vi "PathPlanner_Trajectory_GenerateStates_Pass1.vi"(9 "StartingSpeeds":T5 {"vOmega" format="%10.3f"; "vY" format="%10.3f"; "vX" format="%10.3f"}, 10 "in PathPlannerStates":T1[](array[typedef]) {"TargetHolonomicRotation"."SIN" format="%13.4f"; "TargetHolonomicRotation"."COS" format="%13.4f"; "TargetHolonomicRotation"."VALUE" format="%13.4f"; "Heading"."SIN" format="%13.4f"; "Heading"."COS" format="%13.4f"; "Heading"."VALUE" format="%13.4f"; "PositionMeters"."Y" format="%14.3f"; "PositionMeters"."X" format="%14.3f"}, 11 "PathPlannerPath":T6={"Reversed"=FALSE, "RotationTargets"=[], "ConstraintZones"=[], "EventMarkers"=[], "GlobalConstraints"={"MaxVelocityMps;"=0.0, "MaxAccelerationMpsSq;"=0.0, "MaxAngularVelRadPsEc;"=0.0, "MaxAngularAccRadPSecSq"=0.0, "Exists"=FALSE, "Unlimited"=FALSE, "NominalVoltageVolts"=12.0}, "GoalEndState"={"VelocityMPS"=0.0, "Rotation"={"VALUE"=0.0, "COS"=1.0, "SIN"=0.0}}, "AllPoints"=[], "Name"="", "Waypoints"=[], "PointTowardsZones"=[], "IdealStartingState"={"VelocityMPS"=0.0, "Rotation"={"VALUE"=1.0, "COS"=0.0, "SIN"=0.0}}, "IsChoreoPath"=FALSE, "PreventFlipping"=FALSE} {"IdealStartingState"."Rotation"."SIN" format="%13.4f"; "IdealStartingState"."Rotation"."COS" format="%13.4f"; "IdealStartingState"."Rotation"."VALUE" format="%13.4f"; "PointTowardsZones"."TargetPosition"."Y" format="%14.3f"; "PointTowardsZones"."TargetPosition"."X" format="%14.3f"; "PointTowardsZones"."RotationOffset"."SIN" format="%13.4f"; "PointTowardsZones"."RotationOffset"."COS" format="%13.4f"; "PointTowardsZones"."RotationOffset"."VALUE" format="%13.4f"; "Waypoints"."nextControl"."Y" format="%14.3f"; "Waypoints"."nextControl"."X" format="%14.3f"; "Waypoints"."anchor"."Y" format="%14.3f"; "Waypoints"."anchor"."X" format="%14.3f"; "Waypoints"."prevControl"."Y" format="%14.3f"; "Waypoints"."prevControl"."X" format="%14.3f"; "AllPoints"."RotationTarget"."rotation"."SIN" format="%13.4f"; "AllPoints"."RotationTarget"."rotation"."COS" format="%13.4f"; "AllPoints"."RotationTarget"."rotation"."VALUE" format="%13.4f"; "AllPoints"."Position"."Y" format="%14.3f"; "AllPoints"."Position"."X" format="%14.3f"; "GoalEndState"."Rotation"."SIN" format="%13.4f"; "GoalEndState"."Rotation"."COS" format="%13.4f"; "GoalEndState"."Rotation"."VALUE" format="%13.4f"; "RotationTargets"."rotation"."SIN" format="%13.4f"; "RotationTargets"."rotation"."COS" format="%13.4f"; "RotationTargets"."rotation"."VALUE" format="%13.4f"}) -> (3 "out PathPlannerStates":T1[](array[typedef]) {"TargetHolonomicRotation"."SIN" format="%13.4f"; "TargetHolonomicRotation"."COS" format="%13.4f"; "TargetHolonomicRotation"."VALUE" format="%13.4f"; "Heading"."SIN" format="%13.4f"; "Heading"."COS" format="%13.4f"; "Heading"."VALUE" format="%13.4f"; "PositionMeters"."Y" format="%14.3f"; "PositionMeters"."X" format="%14.3f"})   [LabVIEW 2019, in "PathPlanner24.lvlib"]
doc: "Internal routine to help create a trajectory from a path."
uses:
  PathPlanner24.lvlib
  TypeDef/PathPlannerTrajectoryState.ctl
  <vilib>/Rock Robotics/WPI/ThirdParty/JAS_Junk/TrajLib/TypeDef/TRANSLATION2D.ctl
  <vilib>/Rock Robotics/WPI/ThirdParty/JAS_Junk/TrajLib/TypeDef/ROTATION2D.ctl
  TypeDef/PathPlannerPathConstraints.ctl
  TypeDef/PathPlannerPath.ctl
  TypeDef/PathPlannerRotationTarget.ctl
  TypeDef/PathPlannerConstraintsZone.ctl
  TypeDef/PathPlannerEventMarker.ctl
  TypeDef/PathPlannerCommandUtil.ctl
  ENum/PathPlanner_CommandUtilType_ENUM.ctl
  TypeDef/PathPlannerGoalEndState.ctl
  TypeDef/PathPlannerPathPoint.ctl
  TypeDef/PathPlannerWaypoint.ctl
  TypeDef/PathPlannerPointTowardsZone.ctl
  TypeDef/PathPlannerIdealStartingState.ctl
  <vilib>/Rock Robotics/WPI/ThirdParty/JAS_Junk/TrajLib/TypeDef/CHASSIS_SPEEDS.ctl
  PathPlanner_GeomUtil_CalculateRadius.vi
  <vilib>/Rock Robotics/WPI/ThirdParty/JAS_Junk/TrajLib/Translation2d_Create.vi
  <vilib>/Rock Robotics/WPI/ThirdParty/JAS_Junk/TrajLib/Translation2d_GetXY.vi
  <vilib>/Rock Robotics/WPI/ThirdParty/JAS_Junk/TrajLib/Rotation2d_CreateXY.vi
  <vilib>/Rock Robotics/WPI/ThirdParty/JAS_Junk/TrajLib/Translation2d_GetDistance.vi
  <vilib>/Rock Robotics/WPI/ThirdParty/JAS_Junk/TrajLib/Trajectory_Library.lvlib
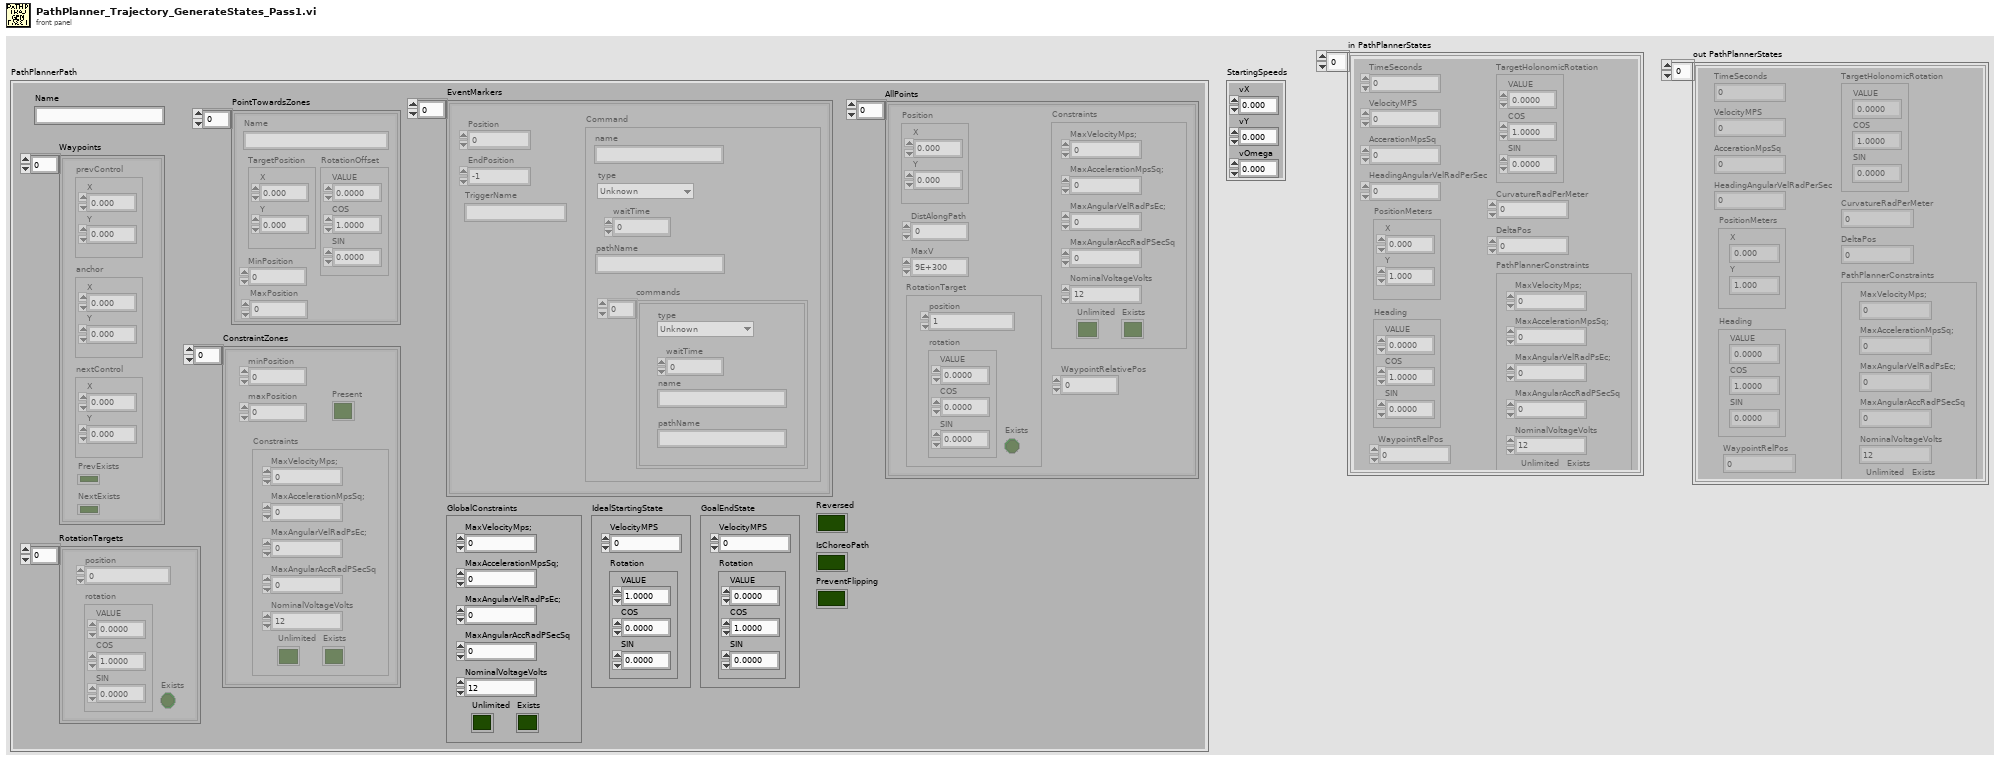
[diagram p1: front panel]
types:
  T1 = typedef "PathPlanner24.lvlib/PathPlannerTrajectoryState.ctl" = cluster{"TimeSeconds":dbl, "VelocityMPS":dbl, "AccerationMpsSq":dbl, "HeadingAngularVelRadPerSec":dbl, "PositionMeters":T2, "Heading":T3, "TargetHolonomicRotation":T3, "CurvatureRadPerMeter":dbl, "PathPlannerConstraints":T4, "DeltaPos":dbl, "WaypointRelPos":dbl}
  T2 = typedef "Trajectory_Library.lvlib/TRANSLATION2D.ctl" = cluster{"X":dbl, "Y":dbl}
  T3 = typedef "Trajectory_Library.lvlib/ROTATION2D.ctl" = cluster{"VALUE":dbl, "COS":dbl, "SIN":dbl}
  T4 = typedef "PathPlanner24.lvlib/PathPlannerPathConstraints.ctl" = cluster{"MaxVelocityMps;":dbl, "MaxAccelerationMpsSq;":dbl, "MaxAngularVelRadPsEc;":dbl, "MaxAngularAccRadPSecSq":dbl, "Exists":bool, "Unlimited":bool, "NominalVoltageVolts":dbl}
  T5 = typedef "Trajectory_Library.lvlib/CHASSIS_SPEEDS.ctl" = cluster{"vX":dbl, "vY":dbl, "vOmega":dbl}
  T6 = typedef "PathPlanner24.lvlib/PathPlannerPath.ctl" = cluster{"Reversed":bool, "RotationTargets":T7[], "ConstraintZones":T8[], "EventMarkers":T9[], "GlobalConstraints":T4, "GoalEndState":T12, "AllPoints":T13[], "Name":string, "Waypoints":T14[], "PointTowardsZones":T15[], "IdealStartingState":T16, "IsChoreoPath":bool, "PreventFlipping":bool}
  T7 = typedef "PathPlanner24.lvlib/PathPlannerRotationTarget.ctl" = cluster{"position":dbl, "rotation":T3, "Exists":bool}
  T8 = typedef "PathPlanner24.lvlib/PathPlannerConstraintsZone.ctl" = cluster{"minPosition":dbl, "maxPosition":dbl, "Constraints":T4, "Present":bool}
  T9 = typedef "PathPlanner24.lvlib/PathPlannerEventMarker.ctl" = cluster{"Position":dbl, "Command":T10, "TriggerName":string, "EndPosition":dbl}
  T10 = typedef "PathPlanner24.lvlib/PathPlannerCommandUtil.ctl" = cluster{"waitTime":dbl, "name":string, "pathName":string, "commands":cluster{"type":T11, "waitTime":dbl, "name":string, "pathName":string}[], "type":T11}
  T11 = typedef "PathPlanner24.lvlib/PathPlanner_CommandUtilType_ENUM.ctl" = enum16{"Unknown", "Wait", "Named", "Path", "Sequential", "Parallel", "Race", "Deadline"}
  T12 = typedef "PathPlanner24.lvlib/PathPlannerGoalEndState.ctl" = cluster{"VelocityMPS":dbl, "Rotation":T3}
  T13 = typedef "PathPlanner24.lvlib/PathPlannerPathPoint.ctl" = cluster{"Position":T2, "DistAlongPath":dbl, "MaxV":dbl, "Constraints":T4, "RotationTarget":T7, "WaypointRelativePos":dbl}
  T14 = typedef "PathPlanner24.lvlib/PathPlannerWaypoint.ctl" = cluster{"prevControl":T2, "anchor":T2, "nextControl":T2, "PrevExists":bool, "NextExists":bool}
  T15 = typedef "PathPlanner24.lvlib/PathPlannerPointTowardsZone.ctl" = cluster{"RotationOffset":T3, "Name":string, "TargetPosition":T2, "MinPosition":dbl, "MaxPosition":dbl}
  T16 = typedef "PathPlanner24.lvlib/PathPlannerIdealStartingState.ctl" = cluster{"VelocityMPS":dbl, "Rotation":T3}
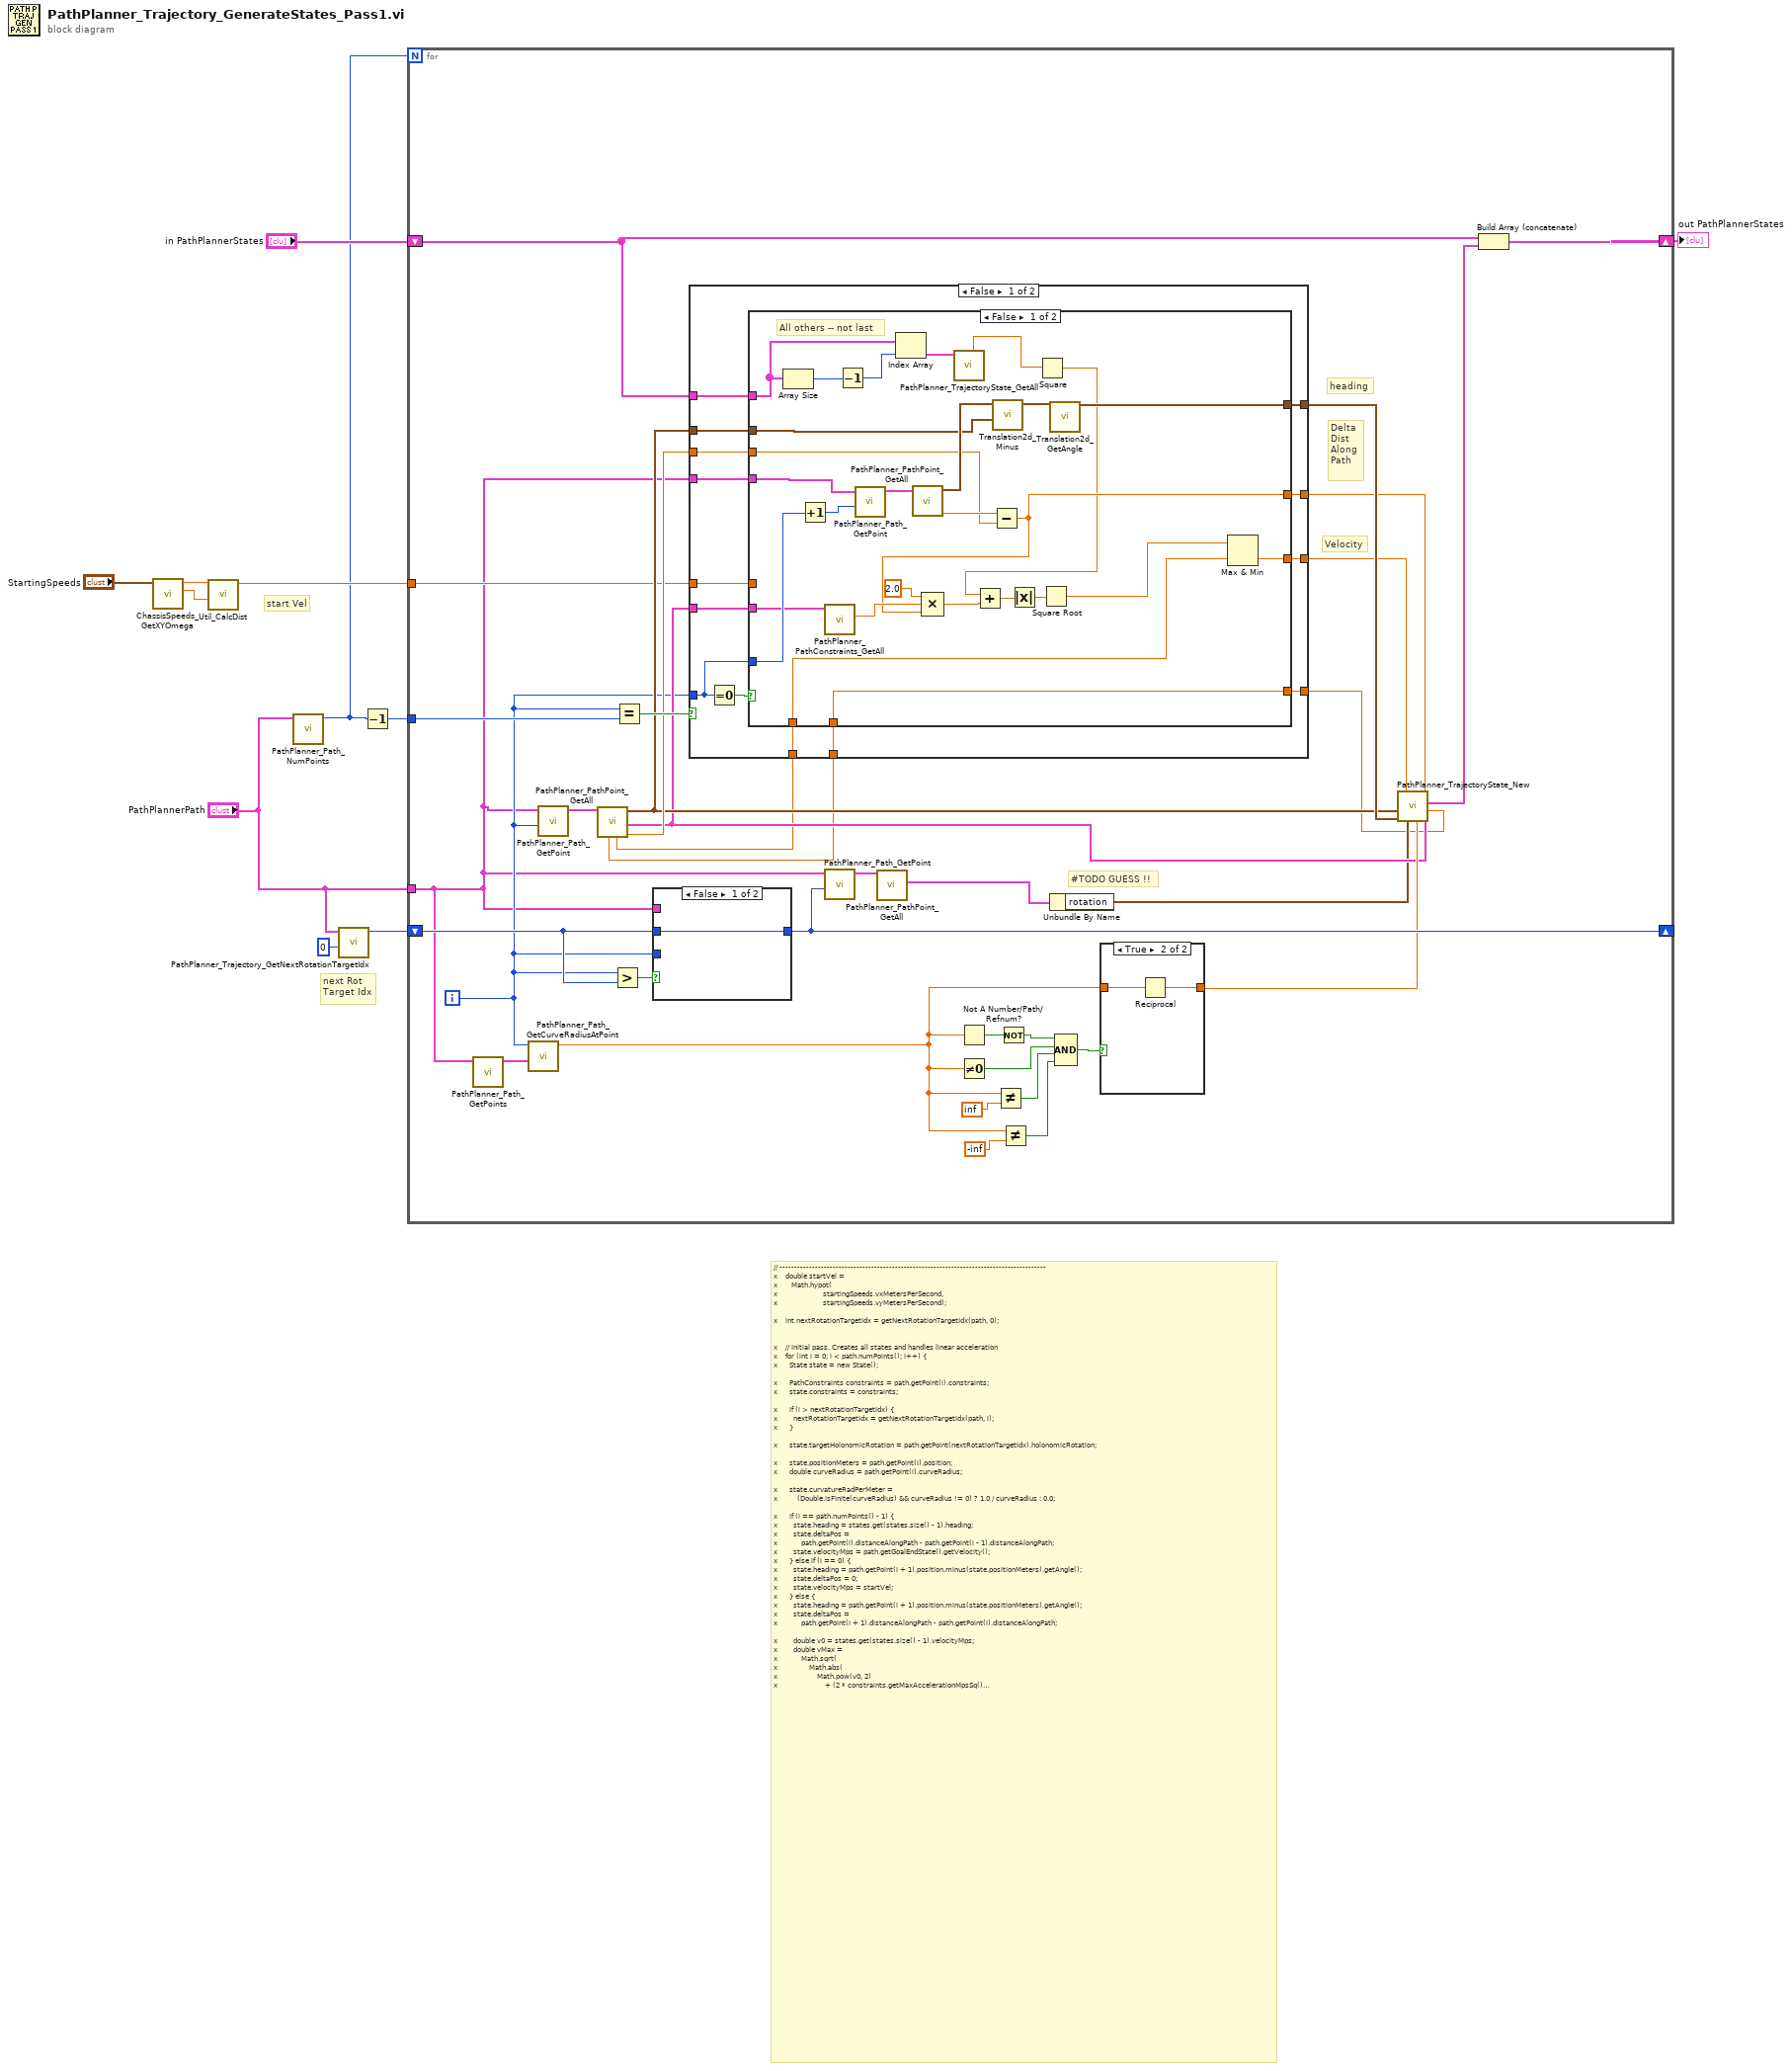
[diagram p0: block diagram]
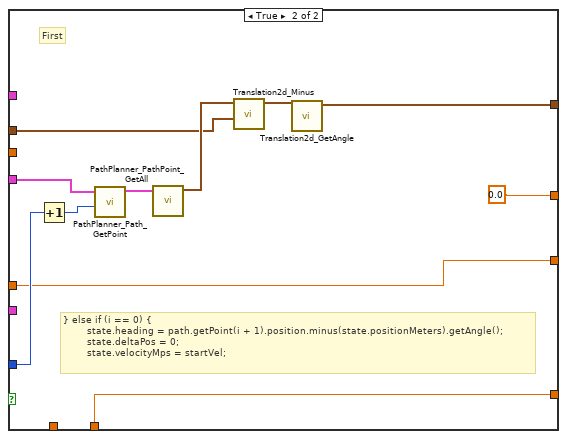
[diagram p2: hidden frame]
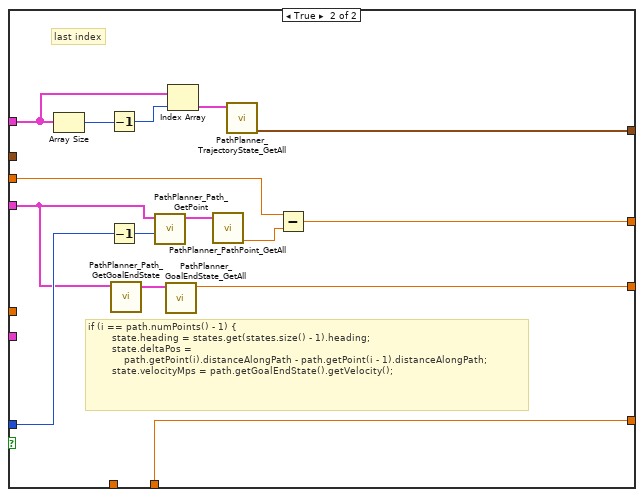
[diagram p3: hidden frame]
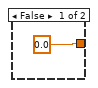
[diagram p4: hidden frame]
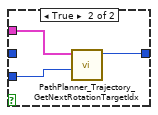
[diagram p5: hidden frame]
diagram:
  # "next Rot\nTarget Idx"
  # "start Vel"
  # "// ------------------------------------------------------------------------------------------\nx    double startVel =\nx       Math.hypot(  \nx                       startingSpeeds.vxMetersPerSecond, \nx                       startingSpeeds.vyMetersPerSecond);\n\nx    int nextRotationTargetIdx = getNextRotationTargetIdx(path, 0);\n\n\nx    // Initial pass. Creates all states and handles linear acceleration\nx    for (int i = 0; i < path.numPoints(); i++) {\nx      State state = new State();\n\nx      PathConstraints constraints = path.getPoint(i).constraints;\nx      state.constraints = constraints;\n\nx      if (i > nextRotationTargetIdx) {\nx        nextRotationTargetIdx = getNextRotationTargetIdx(path, i);\nx      }\n\nx      state.targetHolonomicRotation = path.getPoint(nextRotationTargetIdx).holonomicRotation;\n\nx      state.positionMeters = path.getPoint(i).position;\nx      double curveRadius = path.getPoint(i).curveRadius;\n\nx      state.curvatureRadPerMeter =\nx          (Double.isFinite(curveRadius) && curveRadius != 0) ? 1.0 / curveRadius : 0.0;\n\nx      if (i == path.numPoints() - 1) {\nx        state.heading = states.get(states.size() - 1).heading;\nx        state.deltaPos =\nx            path.getPoint(i).distanceAlongPath - path.getPoint(i - 1).distanceAlongPath;\nx        state.velocityMps = path.getGoalEndState().getVelocity();\nx      } else if (i == 0) {\nx        state.heading = path.getPoint(i + 1).position.minus(state.positionMeters).getAngle();\nx        state.deltaPos = 0;\nx        state.velocityMps = startVel;\nx      } else {\nx        state.heading = path.getPoint(i + 1).position.minus(state.positionMeters).getAngle();\nx        state.deltaPos =\nx            path.getPoint(i + 1).distanceAlongPath - path.getPoint(i).distanceAlongPath;\n\nx        double v0 = states.get(states.size() - 1).velocityMps;\nx        double vMax =\nx            Math.sqrt(\nx                Math.abs(\nx                    Math.pow(v0, 2)\nx                        + (2 * constraints.getMaxAccelerationMpsSq() * state.deltaPos)));\nx        state.velocityMps = Math.min(vMax, path.getPoint(i).maxV);\n      }\n\nX      states.add(state);\n    }"
  n1 = call <vilib>:"ChassisSpeeds_GetXYOmega.vi"("CHASSIS"="StartingSpeeds") -> ("vY"=w5:dbl, "vX"=w6:dbl)  [unwired: 8 in, 1 out]
  n2 = call <vilib>:"Util_CalcDist.vi"("Y"=w5, "X"=w6) -> ("DIST"=w4:dbl)  [unwired: 9 in]
  n3 = call "PathPlanner_Path_NumPoints.vi"("PathPlannerPath"="PathPlannerPath") -> ("NumPoints"=w1:i32)  [unwired: 10 in]
  n4 = call "PathPlanner_Trajectory_GetNextRotationTargetIdx.vi"("Starting Index"=0, "PathPlannerPath"="PathPlannerPath") -> ("Idx"=w8:i32)  [unwired: 8 in, 1 out]
  n5 = Decrement(x=w1) -> (x-1=w3:i32)
  n6 = for {
    N: w1 -> [_]
    shift-right: [w46] -> w10
    shift-left: "in PathPlannerStates" -> [w34]
    tunnel: w4 -> [w27]
    shift-right: [w43] -> _
    shift-left: w8 -> [w44]
    tunnel: "PathPlannerPath" -> [w14]
    tunnel: w3 -> [w36]
    i -> [w16]
    # "#TODO GUESS !!"
    # "Velocity"
    # "Delta\nDist\nAlong\nPath"
    # "heading"
    n7 = call "PathPlanner_Path_GetPoints.vi"("PathPlannerPath"=w14) -> ("Points"=w15:T13[])  [unwired: 10 in]
    n8 = call "PathPlanner_Path_GetCurveRadiusAtPoint.vi"("Points"=w15, "Index"=w16) -> ("Radius"=w17:dbl)  [unwired: 9 in]
    n9 = call "PathPlanner_Path_GetPoint.vi"("Index"=w16, "PathPlannerPath"=w14) -> ("Point"=w25:T13)  [unwired: 9 in]
    n10 = call "PathPlanner_PathPoint_GetAll.vi"("PathPlannerPoint"=w25) -> ("DistAlongPath"=w32:dbl, "Constraints"=w26:T4, "Position"=w28:T2, "MaxV"=w18:dbl, "WaypointRelativePos"=w13:dbl)  [unwired: 5 in, 1 out]
    n11 = Greater?(x=w16, y=w44) -> (0:w45:bool)
    n12 = Equal?(x=w16, y=w36) -> (x = y?=w35:bool)
    n13 = case shown="False" w45 {
      tunnel: w16 -> [_ w120]
      tunnel: w14 -> [_ w119]
      tunnel: [w117 w118] -> w43
      tunnel: w44 -> [w117 _]
      frame False {
      }
      frame True {
        n14 = call "PathPlanner_Trajectory_GetNextRotationTargetIdx.vi"("Starting Index"=w120, "PathPlannerPath"=w119) -> ("Idx"=w118:i32)  [unwired: 8 in, 1 out]
      }
    }
    n15 = case shown="False" w35 {
      tunnel: w16 -> [w59 w108]
      tunnel: w34 -> [w51 w112]
      tunnel: [w56 w109] -> w33
      tunnel: w14 -> [w58 w102]
      tunnel: w32 -> [w52 w104]
      tunnel: [w55 w103] -> w30
      tunnel: [w54 w100] -> w29
      tunnel: w28 -> [w57 _]
      tunnel: w27 -> [w53 _]
      tunnel: w26 -> [w50 _]
      tunnel: w18 -> [w49 _]
      tunnel: w13 -> [w48 w99]
      tunnel: [w47 w99] -> w12
      frame False {
        n16 = Equal To 0?(x=w59) -> (x = 0?=w60:bool)
        n17 = case shown="False" w60 {
          tunnel: w59 -> [w83 w96]
          tunnel: w58 -> [w82 w95]
          tunnel: w57 -> [w81 w92]
          tunnel: [w80 w91] -> w56
          tunnel: [w69 0.0] -> w55
          tunnel: [w64 w89] -> w54
          tunnel: w53 -> [_ w89]
          tunnel: w52 -> [w78 _]
          tunnel: w51 -> [w74 _]
          tunnel: w50 -> [w72 _]
          tunnel: w49 -> [w63 _]
          tunnel: w48 -> [w61 w88]
          tunnel: [w61 w88] -> w47
          frame False {
            # "All others -- not last"
            n18 = Array Size(array=w74) -> (size(s)=w77:i32)
            n19 = Increment(x=w83) -> (x+1=w86:i32)
            n20 = call "PathPlanner_PathConstraints_GetAll.vi"("PathPlannerConstraints"=w72) -> ("MaxAccelerationMpsSq;"=w71:dbl)  [unwired: 6 in, 4 out]
            n21 = Decrement(x=w77) -> (x-1=w76:i32)
            n22 = call "PathPlanner_Path_GetPoint.vi"("Index"=w86, "PathPlannerPath"=w82) -> ("Point"=w87:T13)  [unwired: 9 in]
            n23 = Index Array(array=w74, index=w76) -> (element=w75:T1)
            n24 = call "PathPlanner_PathPoint_GetAll.vi"("PathPlannerPoint"=w87) -> ("DistAlongPath"=w79:dbl, "Position"=w84:T2)  [unwired: 5 in, 4 out]
            n25 = call "PathPlanner_TrajectoryState_GetAll.vi"("PathPlannerState"=w75) -> ("VelocityMPS"=w73:dbl)  [unwired: 1 in, 9 out]
            n26 = Subtract(x=w79, y=w78) -> (x-y=w69:dbl)
            n27 = Compound Arithmetic op=MULTIPLY(2.0 ("x"), w71, w69) -> (w68:dbl)
            n28 = call <vilib>:"Translation2d_Minus.vi"("other Translation"=w81, "In Translation"=w84) -> ("Out Translation"=w85:T2)  [unwired: 9 in]
            n29 = Square(x=w73) -> (x^2=w65:dbl)
            n30 = Add(x=w65, y=w68) -> (x+y=w67:dbl)
            n31 = Absolute Value(x=w67) -> (abs(x)=w66:dbl)
            n32 = Square Root(x=w66) -> (sqrt(x)=w62:dbl)
            n33 = call <vilib>:"Translation2d_GetAngle.vi"("In Translation"=w85) -> ("Angle_Rotation2d"=w80:T3)  [unwired: 10 in]
            n34 = Max & Min(x=w62, y=w63) -> (min(x,y)=w64:dbl)  [unwired: 1 out]
          }
          frame True {
            # "} else if (i == 0) {\n        state.heading = path.getPoint(i + 1).position.minus(state.positionMeters).getAngle();\n        state.deltaPos = 0;\n        state.velocityMps = startVel;"
            # "First"
            n35 = Increment(x=w96) -> (x+1=w97:i32)
            n36 = call "PathPlanner_Path_GetPoint.vi"("Index"=w97, "PathPlannerPath"=w95) -> ("Point"=w98:T13)  [unwired: 9 in]
            n37 = call "PathPlanner_PathPoint_GetAll.vi"("PathPlannerPoint"=w98) -> ("Position"=w93:T2)  [unwired: 5 in, 5 out]
            n38 = call <vilib>:"Translation2d_Minus.vi"("other Translation"=w92, "In Translation"=w93) -> ("Out Translation"=w94:T2)  [unwired: 9 in]
            n39 = call <vilib>:"Translation2d_GetAngle.vi"("In Translation"=w94) -> ("Angle_Rotation2d"=w91:T3)  [unwired: 10 in]
          }
        }
      }
      frame True {
        # "if (i == path.numPoints() - 1) {\n        state.heading = states.get(states.size() - 1).heading;\n        state.deltaPos =\n            path.getPoint(i).distanceAlongPath - path.getPoint(i - 1).distanceAlongPath;\n        state.velocityMps = path.getGoalEndState().getVelocity();"
        # "last index"
        n40 = Array Size(array=w112) -> (size(s)=w113:i32)
        n41 = Decrement(x=w113) -> (x-1=w111:i32)
        n42 = Decrement(x=w108) -> (x-1=w107:i32)
        n43 = call "PathPlanner_Path_GetGoalEndState.vi"("PathPlannerPath"=w102) -> ("GoalEndState"=w101:T12)  [unwired: 10 in]
        n44 = call "PathPlanner_Path_GetPoint.vi"("Index"=w107, "PathPlannerPath"=w102) -> ("Point"=w106:T13)  [unwired: 9 in]
        n45 = call "PathPlanner_GoalEndState_GetAll.vi"("GoalEndState"=w101) -> ("VelocityMPS"=w100:dbl)  [unwired: 9 in, 1 out]
        n46 = Index Array(array=w112, index=w111) -> (element=w110:T1)
        n47 = call "PathPlanner_PathPoint_GetAll.vi"("PathPlannerPoint"=w106) -> ("DistAlongPath"=w105:dbl)  [unwired: 5 in, 5 out]
        n48 = call "PathPlanner_TrajectoryState_GetAll.vi"("PathPlannerState"=w110) -> ("Heading"=w109:T3)  [unwired: 1 in, 9 out]
        n49 = Subtract(x=w104, y=w105) -> (x-y=w103:dbl)
      }
    }
    n50 = call "PathPlanner_Path_GetPoint.vi"("Index"=w43, "PathPlannerPath"=w14) -> ("Point"=w42:T13)  [unwired: 9 in]
    n51 = call "PathPlanner_PathPoint_GetAll.vi"("PathPlannerPoint"=w42) -> ("RotationTarget"=w20:T7)  [unwired: 5 in, 5 out]
    n52 = Not A Number/Path/Refnum?(number/path/refnum=w17) -> (NaN/Path/Refnum?=w41:bool)
    n53 = Not Equal To 0?(x=w17) -> (x != 0?=w39:bool)
    n54 = Not Equal?(x=w17, y=inf) -> (x != y?=w22:bool)
    n55 = Not(x=w41) -> (.not. x?=w40:bool)
    n56 = Not Equal?(x=w17, y=-inf) -> (x != y?=w21:bool)
    n57 = Unbundle By Name(w20) -> ("rotation"=w19:T3)
    n58 = Compound Arithmetic op=AND(w40, w39, w22, w21) -> (w38:bool)
    n59 = case shown="True" w38 {
      tunnel: w17 -> [_ w116]
      tunnel: [0.0 w115] -> w37
      frame False {
      }
      frame True {
        n60 = Reciprocal(x=w116) -> (1/x=w115:dbl)
      }
    }
    n61 = call "PathPlanner_TrajectoryState_New.vi"("PathPlannerConstraints"=w26, "WaypointRelPos"=w12, "DeltaPos"=w30, "CurvatureRadPerMeter"=w37, "TargetHolonomicRotation"=w19, "VelocityMPS"=w29, "Heading"=w33, "PositionMeters"=w28) -> ("PathPlannerState"=w31:T1)  [unwired: 3 in]
    n62 = Build Array (concatenate)(w34, w31) -> (w46:T1[])
  }
  "out PathPlannerStates" <- w10
